vi "Begin Cheeto.vi"(8 "error in":errorcluster) -> (0 "error out":errorcluster)   [LabVIEW 2016]
doc: "Called before other user functions, this VI is expected to open initial I/O refnums, load in file data, and do all program initialization. Notice that the <B>error out</B> terminal is simply used for data flow. Wiring it to other structures or subVIs ensures that this VI runs first."
uses:
  <vilib>/Rock Robotics/WPI/DriverStation/WPI_DriverStationRobotMode2.ctl
  <vilib>/Rock Robotics/SystemInterfaces/DIO/FPGA_DIOChannel.ctl
  <vilib>/Rock Robotics/WPI/Encoder/WPI_EncoderType.ctl
  <vilib>/Rock Robotics/WPI/ThirdParty/CanMotor/TalonSRX/WPI_CANTalonSRX_APIControlMode.ctl
  <vilib>/Rock Robotics/SystemInterfaces/DIO/FPGA_DIOPWMChannel.ctl
  Robot Global Data.vi
  <vilib>/Rock Robotics/WPI/Counter/WPI_CounterDigitalInputToDigitalSource.vi
  <vilib>/Rock Robotics/WPI/MotorControl/WPI_MotorControlOpen Talon.vi
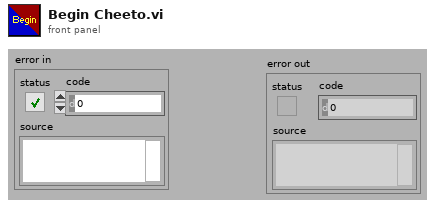
[diagram p1: front panel]
types:
  T1 = typedef "FPGA_DIOPWMChannel.ctl" = enum8{"PWM 0", "PWM 1", "PWM 2", "PWM 3", "PWM 4", "PWM 5", "PWM 6", "PWM 7", "PWM 8", "PWM 9", "PWM MXP 0", "PWM MXP 1", "PWM MXP 2", "PWM MXP 3", "PWM MXP 4", "PWM MXP 5", "PWM MXP 6", "PWM MXP 7", "PWM MXP 8", "PWM MXP 9", "Invalid"}
  T2 = typedef "WPI_CANTalonSRX_APIControlMode.ctl" = enum8{"Percent VBus", "Speed", "Position", "Slave", "Unchanged / Invalid", "Voltage Compensation", "Current", "Motion Profile", "Motion Magic"}
  T3 = typedef "WPI_EncoderType.ctl" = enum16{"1x", "2x", "4x"}
  T4 = typedef "FPGA_DIOChannel.ctl" = enum8{"DIO 0", "DIO 1", "DIO 2", "DIO 3", "DIO 4", "DIO 5", "DIO 6", "DIO 7", "DIO 8", "DIO 9", "DIO MXP 0", "DIO MXP 1", "DIO MXP 2", "DIO MXP 3", "DIO MXP 4", "DIO MXP 5", "DIO MXP 6", "DIO MXP 7", "DIO MXP 8", "DIO MXP 9", "DIO MXP 10", "DIO MXP 11", "DIO MXP 12", "DIO MXP 13", "DIO MXP 14", "DIO MXP 15", "SPI Port CS1", "SPI Port CS2", "SPI Port CS3", "SPI Port MISO", "SPI Port MOSI", "Invalid"}
  T5 = typedef "WPI_DriverStationRobotMode2.ctl" = enum16{"Autonomous Disabled", "Autonomous Enabled", "Teleop Disabled", "Teleop Enabled", "Disconnected", "Finish", "Test Disabled", "Test Enabled", "Emergency Stopped"}
  T6 = typedef "WPI_MotorControlDeviceRef.ctl" = cluster{"DeviceStatus":errorcluster, "Type":T7, "PWM":cluster{"PWM Channel":T1, "DeadBand":T8}, "CAN":cluster{"Device Number":u8, "SetOutput VI Ref":variant, "GetOutput VI Ref":variant, "Enable VI Ref":variant, "Disable VI Ref":variant, "Data":variant}, "Invert":bool}
  T7 = typedef "WPI_MotorControlType.ctl" = enum16{"PWM", "CAN"}
  T8 = typedef "WPI_PWMDeadband.ctl" = cluster{"Name":string, "maxPositivePwm":i32, "minPositivePwm":i32, "centerPwm":i32, "maxNegativePwm":i32, "minNegativePwm":i32, "angularRange":u16}
  T9 = typedef "WPI_DigitalInputDevRef.ctl" = cluster{"DevStatus":errorcluster, "DIO Channel":T4}
  T10 = typedef "FPGA_CounterEncoderSourceConvertionLVSourceType.ctl" = cluster{"DevStatus":errorcluster, "AnalogTriggerMode?":bool, "DigitalMode":cluster{"DIO Channel":T11}, "AnalogTriggerMode":cluster{"AnalogTriggerIndex":T12, "OutputType":T13}}
  T11 = typedef "FPGA_DIODigitalSourceChannel.ctl" = enum8{"DIO 0", "DIO 1", "DIO 2", "DIO 3", "DIO 4", "DIO 5", "DIO 6", "DIO 7", "DIO 8", "DIO 9", "DIO MXP 0", "DIO MXP 1", "DIO MXP 2", "DIO MXP 3", "DIO MXP 4", "DIO MXP 5", "DIO MXP 6", "DIO MXP 7", "DIO MXP 8", "DIO MXP 9", "DIO MXP 10", "DIO MXP 11", "DIO MXP 12", "DIO MXP 13", "DIO MXP 14", "DIO MXP 15", "Disabled"}
  T12 = typedef "FPGA_AnalogTriggerIndex.ctl" = enum8{"Trig 0", "Trig 1", "Trig 2", "Trig 3", "Trig 4", "Trig 5", "Trig 6", "Trig 7", "Invalid"}
  T13 = typedef "FPGA_AnalogTriggerOutType.ctl" = enum16{"InWindow", "TriggerState", "Rising", "Falling"}
  T14 = typedef "WPI_EncoderDevRef.ctl" = cluster{"DevStatus":errorcluster, "EncoderIndex":T15, "CounterIndex":T16, "DistancePerCount":dbl, "Decoding Type":T3}
  T15 = typedef "FPGA_EncoderIdx.ctl" = enum8{"Enc 0", "Enc 1", "Enc 2", "Enc 3", "Enc 4", "Enc 5", "Enc 6", "Enc 7", "Invalid"}
  T16 = typedef "FPGA_CounterCtrSystemIndex.ctl" = enum8{"Ctr 0", "Ctr 1", "Ctr 2", "Ctr 3", "Ctr 4", "Ctr 5", "Ctr 6", "Ctr 7", "Invalid"}
  T17 = typedef "WPI_ServoDeviceRef.ctl" = cluster{"DeviceStatus":errorcluster, "PWM Channel":T1, "DeadBand":T8}
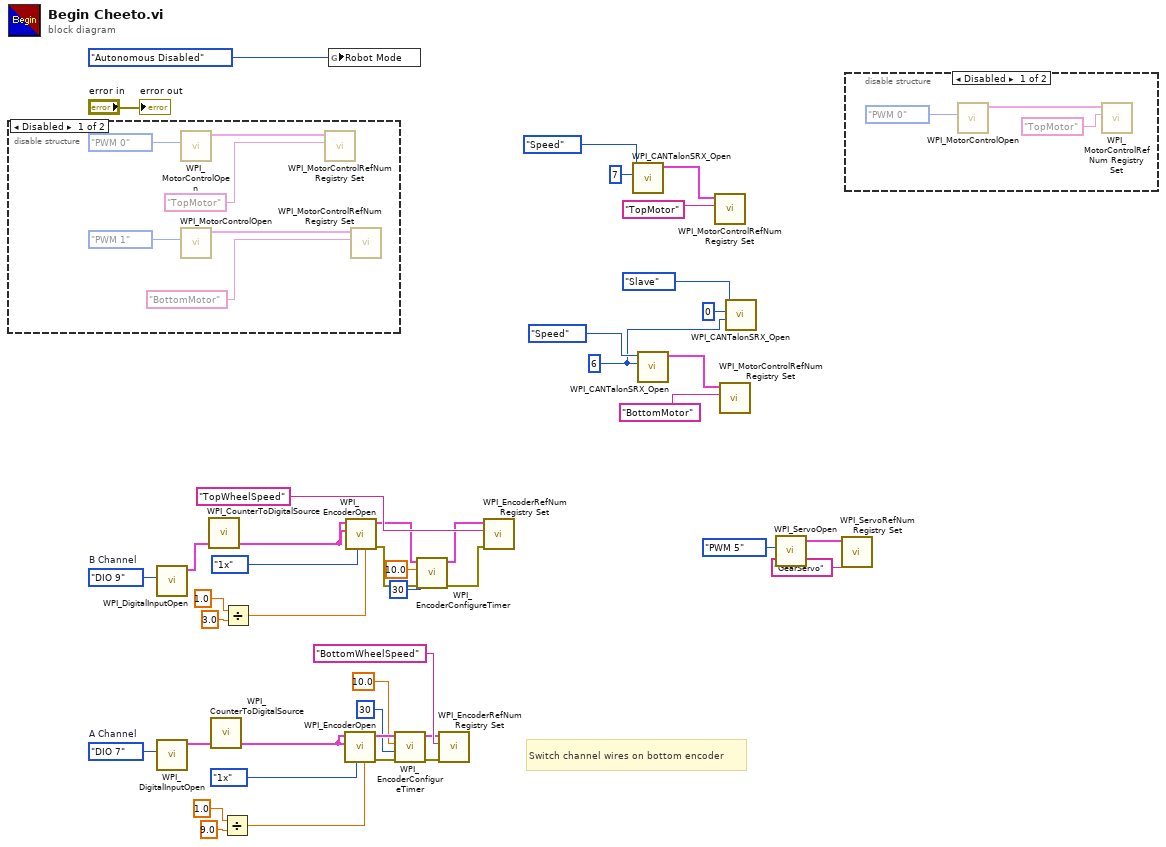
[diagram p0: block diagram]
diagram:
  w10 = u8 6 ("Device Number")
  w34 = FPGA_DIOChannel."DIO 7"  # A Channel
  w41 = FPGA_DIOChannel."DIO 9"  # B Channel
  # "Switch channel wires on bottom encoder"
  n1 = disable-structure shown="Disabled" {
    frame Disabled {
      n2 = call-poly <vilib>:"WPI_MotorControlOpen.vi"("PWM Channel"=FPGA_DIOPWMChannel."PWM 0") -> ("MotorControlDeviceRef"=w49:T6)  [unwired: 9 in, 1 out]
      n3 = call-poly <vilib>:"WPI_MotorControlOpen.vi"("PWM Channel"=FPGA_DIOPWMChannel."PWM 1") -> ("MotorControlDeviceRef"=w45:T6)  [unwired: 9 in, 1 out]
      n4 = call <vilib>:"WPI_MotorControlRefNum Registry Set.vi"("refnum name"="TopMotor", "MotorControlDevRef"=w49) -> ()  [unwired: 8 in, 2 out]
      n5 = call <vilib>:"WPI_MotorControlRefNum Registry Set.vi"("refnum name"="BottomMotor", "MotorControlDevRef"=w45) -> ()  [unwired: 8 in, 2 out]
    }
    frame Enabled {
    }
  }
  n6 = call <vilib>:"WPI_DigitalInputOpen.vi"("DIO Channel"=w41) -> ("DigitalInputDevRef"=w40:T9)  [unwired: 1 in, 9 out]
  n7 = call <vilib>:"WPI_DigitalInputOpen.vi"("DIO Channel"=w34) -> ("DigitalInputDevRef"=w35:T9)  [unwired: 1 in, 9 out]
  n8 = call-poly <vilib>:"WPI_CounterToDigitalSource.vi"("DigitalInputDevRef"=w40) -> ("Digital Source"=w20:T10)  [unwired: 6 out]
  n9 = call-poly <vilib>:"WPI_CounterToDigitalSource.vi"("DigitalInputDevRef"=w35) -> ("Digital Source"=w21:T10)  [unwired: 6 out]
  n10 = Divide(x=1.0, y=9.0) -> (x/y=w28:dbl)
  n11 = Divide(x=1.0, y=3.0) -> (x/y=w33:dbl)
  n12 = global write "Robot Global Data.vi" "Robot Mode"(WPI_DriverStationRobotMode2."Autonomous Disabled" ("Robot Mode")) -> ()
  n13 = call <vilib>:"WPI_EncoderOpen.vi"("DistancePerCount"=w28, "Decoding Type"=WPI_EncoderType."1x", "BSource"=w21, "ASource"=w21) -> ("error out"=w22:errorcluster, "EncoderDevRef"=w25:T14)  [unwired: 4 in, 2 out]
  n14 = call <vilib>:"WPI_EncoderOpen.vi"("DistancePerCount"=w33, "Decoding Type"=WPI_EncoderType."1x", "BSource"=w20, "ASource"=w20) -> ("error out"=w16:errorcluster, "EncoderDevRef"=w19:T14)  [unwired: 4 in, 2 out]
  n15 = call <vilib>:"WPI_EncoderConfigureTimer.vi"("error in (no error)"=w22, "Number Samples to Average"=u8 30, "Minimum Rate"=10.0, "EncoderDevRef"=w25) -> ("error out"=w26:errorcluster, "EncoderDevRef"=w27:T14)  [unwired: 6 in]
  n16 = call <vilib>:"WPI_EncoderConfigureTimer.vi"("error in (no error)"=w16, "Number Samples to Average"=u8 30, "Minimum Rate"=10.0, "EncoderDevRef"=w19) -> ("error out"=w17:errorcluster, "EncoderDevRef"=w18:T14)  [unwired: 6 in]
  n17 = call <vilib>:"WPI_EncoderRefNum Registry Set.vi"("error in (no error)"=w26, "refnum name"="BottomWheelSpeed", "EncoderDevRef"=w27) -> ()  [unwired: 7 in, 2 out]
  n18 = call <vilib>:"WPI_EncoderRefNum Registry Set.vi"("error in (no error)"=w17, "refnum name"="TopWheelSpeed", "EncoderDevRef"=w18) -> ()  [unwired: 7 in, 2 out]
  n19 = call <vilib>:"WPI_CANTalonSRX_Open.vi"("Device Number"=u8 7, "Control Mode"=WPI_CANTalonSRX_APIControlMode."Speed") -> ("CAN Talon SRX Ref"=w4:T6)  [unwired: 8 in, 1 out]
  n20 = call <vilib>:"WPI_CANTalonSRX_Open.vi"("Device Number"=w10, "Control Mode"=WPI_CANTalonSRX_APIControlMode."Speed") -> ("CAN Talon SRX Ref"=w13:T6)  [unwired: 8 in, 1 out]
  n21 = call <vilib>:"WPI_MotorControlRefNum Registry Set.vi"("refnum name"="TopMotor", "MotorControlDevRef"=w4) -> ()  [unwired: 8 in, 2 out]
  n22 = call <vilib>:"WPI_MotorControlRefNum Registry Set.vi"("refnum name"="BottomMotor", "MotorControlDevRef"=w13) -> ()  [unwired: 8 in, 2 out]
  n23 = call <vilib>:"WPI_CANTalonSRX_Open.vi"("Master Device Number"=w10, "Device Number"=u8 0, "Control Mode"=WPI_CANTalonSRX_APIControlMode."Slave") -> ()  [unwired: 7 in, 2 out]
  n24 = call <vilib>:"WPI_ServoOpen.vi"("PWM Channel"=FPGA_DIOPWMChannel."PWM 5") -> ("ServoDeviceRef"=w2:T17)  [unwired: 9 in, 1 out]
  n25 = call <vilib>:"WPI_ServoRefNum Registry Set.vi"("refnum name"="GearServo", "ServoDeviceRef"=w2) -> ()  [unwired: 8 in, 2 out]
  n26 = disable-structure shown="Disabled" {
    frame Disabled {
      n27 = call-poly <vilib>:"WPI_MotorControlOpen.vi"("PWM Channel"=FPGA_DIOPWMChannel."PWM 0") -> ("MotorControlDeviceRef"=w51:T6)  [unwired: 9 in, 1 out]
      n28 = call <vilib>:"WPI_MotorControlRefNum Registry Set.vi"("refnum name"="TopMotor", "MotorControlDevRef"=w51) -> ()  [unwired: 8 in, 2 out]
    }
    frame Enabled {
    }
  }
  "error out" <- "error in"
